vi "Get All Table.vi"(8 "error in (no error)":errorcluster, 11 "SQLObject in":refnum<class "SQLObject.lvclass">) -> (0 "error out":errorcluster, 2 "Result Set":string[][](array[string]), 3 "SQLObject out":refnum<class "SQLObject.lvclass">)   [LabVIEW 2021, in "SQLObject.lvclass"]
uses:
  SQLObject.lvclass
  SQLObject.lvclass/SQLObject.ctl
  <vilib>/JDP Science/JDP Science Common Utilities/Trim Whitespace__JDP.vi
  <vilib>/Utility/Data Type/Get Cluster Information.vi
  <vilib>/Utility/Data Type/Get Type Information.vi
  <vilib>/drjdpowell/SQLite Library/SQL Connection/Execute SQL.vi
  <vilib>/drjdpowell/SQLite Library/SQLite.lvlib
  <vilib>/drjdpowell/SQLite Library/SQL Connection/Connection.lvclass
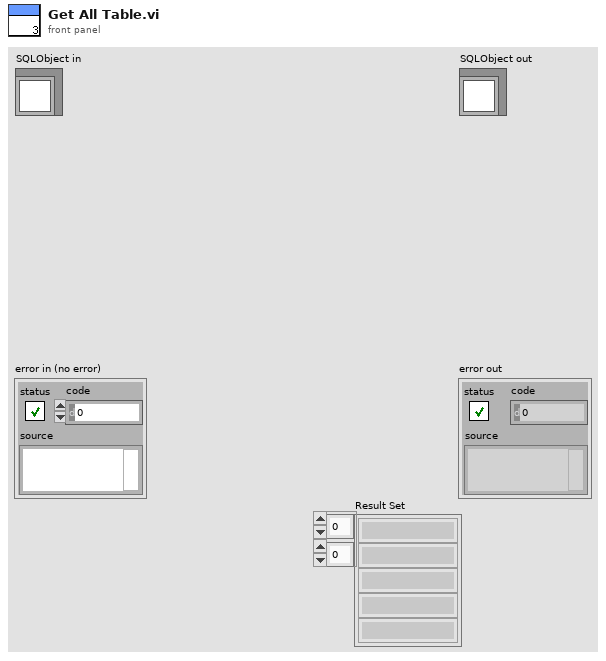
[diagram p1: front panel]
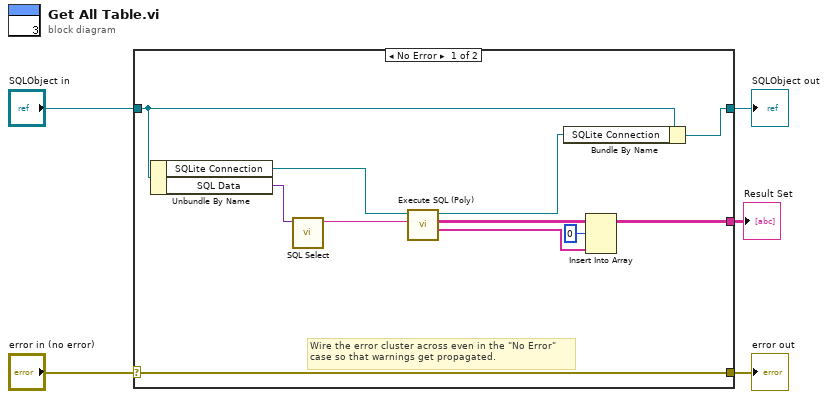
[diagram p0: block diagram]
diagram:
  n1 = case shown="No Error" "error in (no error)" {
    selector: "error in (no error)" -> [w16 w18]
    tunnel: [w16 w18] -> w4
    tunnel: [w6 w17] -> w2
    tunnel: "SQLObject in" -> [w8 w17]
    tunnel: [w12 _] -> w1
    frame No Error {
      # "Wire the error cluster across even in the \"No Error\"\ncase so that warnings get propagated."
      n2 = Unbundle By Name(w8) -> ("SQLite Connection"=w14:refnum<class "Connection.lvclass">, "SQL Data"=w15:variant)
      n3 = call "SQL Select.vi"("variant"=w15) -> ("SQL"=w13:string)  [unwired: 10 in]
      n4 = call-poly <vilib>:"Execute SQL (Poly).vi"("SQL"=w13, "SQLite Connection in"=w14) -> ("Column Names"=w9:string[], "Result Set"=w11:string[][], "SQLite Connection"=w7:refnum<class "Connection.lvclass">)  [unwired: 6 in, 1 out]
      n5 = Bundle By Name(cluster=w8, "SQLite Connection"=w7) -> (w6:refnum<class "SQLObject.lvclass">)
      n6 = Insert Into Array(array=w11, index (row)=0, new element=w9) -> (w12:string[][])  [unwired: 1 in]
    }
    frame Error {
    }
  }
  "error out" <- w4
  "SQLObject out" <- w2
  "Result Set" <- w1
